vi "COMMAND_Status.vi"(8 "error in (no error)":errorcluster, 11 "MH100301DMC in":refnum<class "StageMH100301DMC.lvclass">) -> (0 "error out":errorcluster, 2 "status":T1, 3 "MH100301DMC out":refnum<class "StageMH100301DMC.lvclass">)   [LabVIEW 2010, in "StageMH100301DMC.lvclass"]
uses:
  StageMH100301DMC.lvclass
  status_cluster.ctl
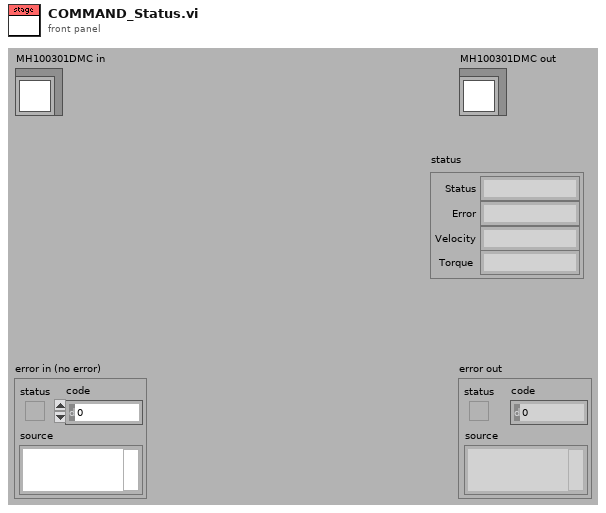
[diagram p1: front panel]
types:
  T1 = typedef "StageMH100301DMC.lvclass/status_cluster.ctl" = cluster{"Status":string, "Torque":string, "Velocity":string, "Error":string}
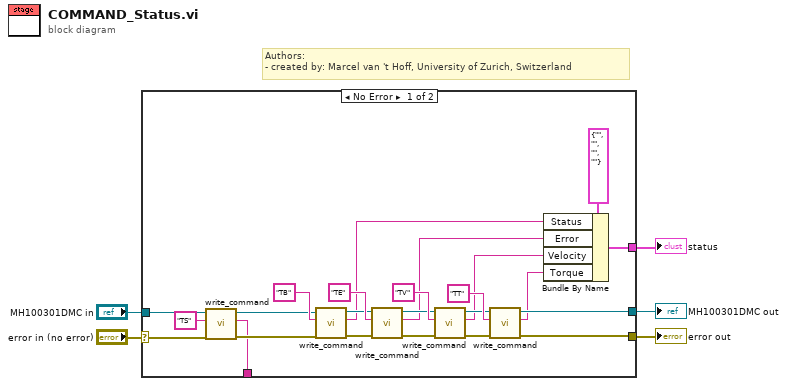
[diagram p0: block diagram]
diagram:
  # "Authors: \n- created by: Marcel van 't Hoff, University of Zurich, Switzerland"
  n1 = case shown="No Error" "error in (no error)" {
    selector: "error in (no error)" -> [w10 w31]
    tunnel: [w16 w31] -> w4
    tunnel: [w17 w30] -> w2
    tunnel: "MH100301DMC in" -> [w11 w30]
    tunnel: [w27 _] -> w1
    tunnel: [w6 _] -> _
    frame No Error {
      n2 = call-dynamic "write_command.vi"("error in (no error)"=w10, "command (without terminating \"\\n\")"="TS" ("command (without terminating \"\\n\")"), "MH100301DMC in"=w11) -> ("error out"=w9:errorcluster, "response out"=w6:string, "MH100301DMC out"=w8:refnum<class "StageMH100301DMC.lvclass">)  [unwired: 6 in]
      n3 = call-dynamic "write_command.vi"("error in (no error)"=w9, "command (without terminating \"\\n\")"="TB" ("command (without terminating \"\\n\")"), "MH100301DMC in"=w8) -> ("error out"=w20:errorcluster, "response out"=w15:string, "MH100301DMC out"=w21:refnum<class "StageMH100301DMC.lvclass">)  [unwired: 6 in]
      n4 = call-dynamic "write_command.vi"("error in (no error)"=w20, "command (without terminating \"\\n\")"="TE" ("command (without terminating \"\\n\")"), "MH100301DMC in"=w21) -> ("error out"=w24:errorcluster, "response out"=w14:string, "MH100301DMC out"=w23:refnum<class "StageMH100301DMC.lvclass">)  [unwired: 6 in]
      n5 = call-dynamic "write_command.vi"("error in (no error)"=w24, "command (without terminating \"\\n\")"="TV" ("command (without terminating \"\\n\")"), "MH100301DMC in"=w23) -> ("error out"=w19:errorcluster, "response out"=w13:string, "MH100301DMC out"=w18:refnum<class "StageMH100301DMC.lvclass">)  [unwired: 6 in]
      n6 = call-dynamic "write_command.vi"("error in (no error)"=w19, "command (without terminating \"\\n\")"="TT" ("command (without terminating \"\\n\")"), "MH100301DMC in"=w18) -> ("error out"=w16:errorcluster, "response out"=w12:string, "MH100301DMC out"=w17:refnum<class "StageMH100301DMC.lvclass">)  [unwired: 6 in]
      n7 = Bundle By Name(cluster=T1 {"Status"="", "Torque"="", "Velocity"="", "Error"=""} ("status"), "Status"=w15, "Error"=w14, "Velocity"=w13, "Torque"=w12) -> (w27:T1)
    }
    frame Error {
    }
  }
  "error out" <- w4
  "MH100301DMC out" <- w2
  "status" <- w1
